vi "LibXML_GetNodeString.vi"(8 "error in":errorcluster, 9 "type":T1(ring), 10 "node":u32) -> (0 "error out":errorcluster, 3 "lvstring":string)   [LabVIEW 2019, in "Tools.lvlib" / "LibXML.lvlib"]
doc: "Gets the XML String of only specific node types (Text, CDATA, or just the values)."
uses:
  LibXML.lvlib
  Error Cluster From Error Code_subroutine.vi
  <vilib>/Utility/error.llb/Trim Whitespace.vi
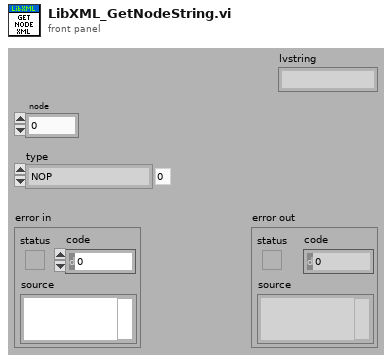
[diagram p1: front panel]
types:
  T1 = enum16{"NOP", "name", "content", "(resolved) content"}
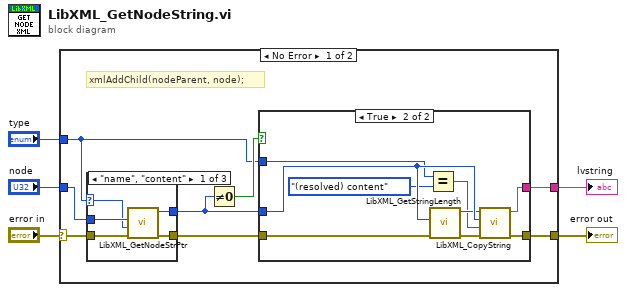
[diagram p0: block diagram]
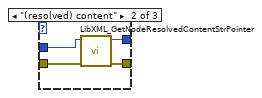
[diagram p2: hidden frame]
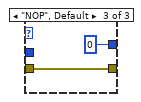
[diagram p3: hidden frame]
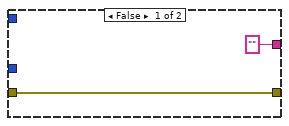
[diagram p4: hidden frame]
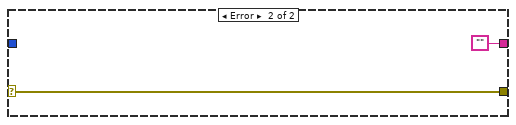
[diagram p5: hidden frame]
diagram:
  n1 = case shown="No Error" "error in" {
    selector: "error in" -> [w12 w37]
    tunnel: [w9 w37] -> w4
    tunnel: "type" -> [w8 _]
    tunnel: "node" -> [w7 _]
    tunnel: [w6 ""] -> w1
    frame No Error {
      # "xmlAddChild(nodeParent, node);"
      n2 = case shown="\"name\", \"content\"" w8 {
        selector: w8 -> [w14 _ _]
        tunnel: [w17 w21 w24] -> w13
        tunnel: w12 -> [w18 w22 w24]
        tunnel: w7 -> [w16 w20 _]
        tunnel: [w15 w19 u32 0] -> w10
        frame "name", "content" {
          n3 = call "LibXML_GetNodeStrPtr.vi"("error in"=w18, "type"=w14, "node"=w16) -> ("error out"=w17:errorcluster, "string ptr  out"=w15:u32)  [unwired: 7 in]
        }
        frame "(resolved) content" {
          n4 = call "LibXML_GetNodeResolvedContentStrPointer.vi"("error in"=w22, "node"=w20) -> ("error out"=w21:errorcluster, "string pointer"=w19:u32)  [unwired: 8 in]
        }
        frame "NOP", Default {
        }
      }
      n5 = Not Equal To 0?(x=w10) -> (x != 0?=w11:bool)
      n6 = case shown="True" w11 {
        tunnel: ["" ("lvstring") w35] -> w6
        tunnel: w13 -> [w26 w34]
        tunnel: w10 -> [_ w32]
        tunnel: [w26 w30] -> w9
        tunnel: w8 -> [_ w29]
        frame False {
        }
        frame True {
          n7 = Equal?(x=w29, y=T1."(resolved) content") -> (x = y?=w27:bool)
          n8 = call "LibXML_GetStringLength.vi"("error in"=w34, "string pointer"=w32) -> ("error out"=w33:errorcluster, "string length"=w31:i32)  [unwired: 4 in]
          n9 = call "LibXML_CopyString.vi"("error in"=w33, "free pointer?"=w27, "string pointer"=w32, "length"=w31) -> ("error out"=w30:errorcluster, "lvstring"=w35:string)  [unwired: 6 in]
        }
      }
    }
    frame Error {
    }
  }
  "error out" <- w4
  "lvstring" <- w1
